vi "Pyro.vi"() -> ()   [LabVIEW 2013]
uses:
  <vilib>/Instr/_visa.llb/VISA Configure Serial Port (Instr).vi
panel:
  out "XY Graph":cluster{dbl[], i32[]}(graph)
  in  "wait":u32
  out "read buffer 3":string
  in  "CUSTOM COMMAND":string(combo)
  in  "Enable Termination\nChar (T)":bool=TRUE
  in  "termination char\n(0xA = '\\n' = LF)":u8=10 format="%.0x"
  in  "timeout (10sec)":u32=10000
  in  "flow control (0:none)":u16(ring) items=["None", "XON/XOFF", "RTS/CTS", "XON/XOFF & RTS/CTS", "DTR/DSR", "XON/XOFF & DTR/DSR"]
  in  "stop bits (10: 1 bit)":u16(ring)=10 items=["1.0"=10, "1.5"=15, "2.0"=20]
  in  "data bits (8)":u16=8 min=5 max=8 step=1
  in  "parity (0:none)":enum16{"None", "Odd", "Even", "Mark", "Space"}(ring)=enum."Even"
  in  "baud rate (9600)":u32=19200
  in  "VISA resource name":refnum<visa-resource-name>="COM3"
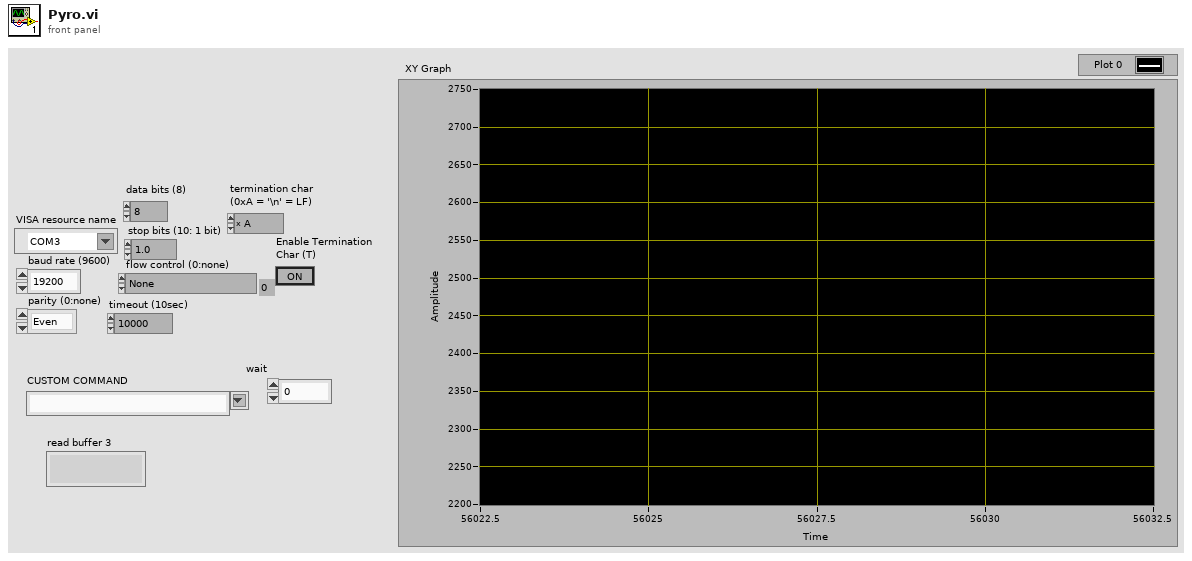
[diagram p1: front panel]
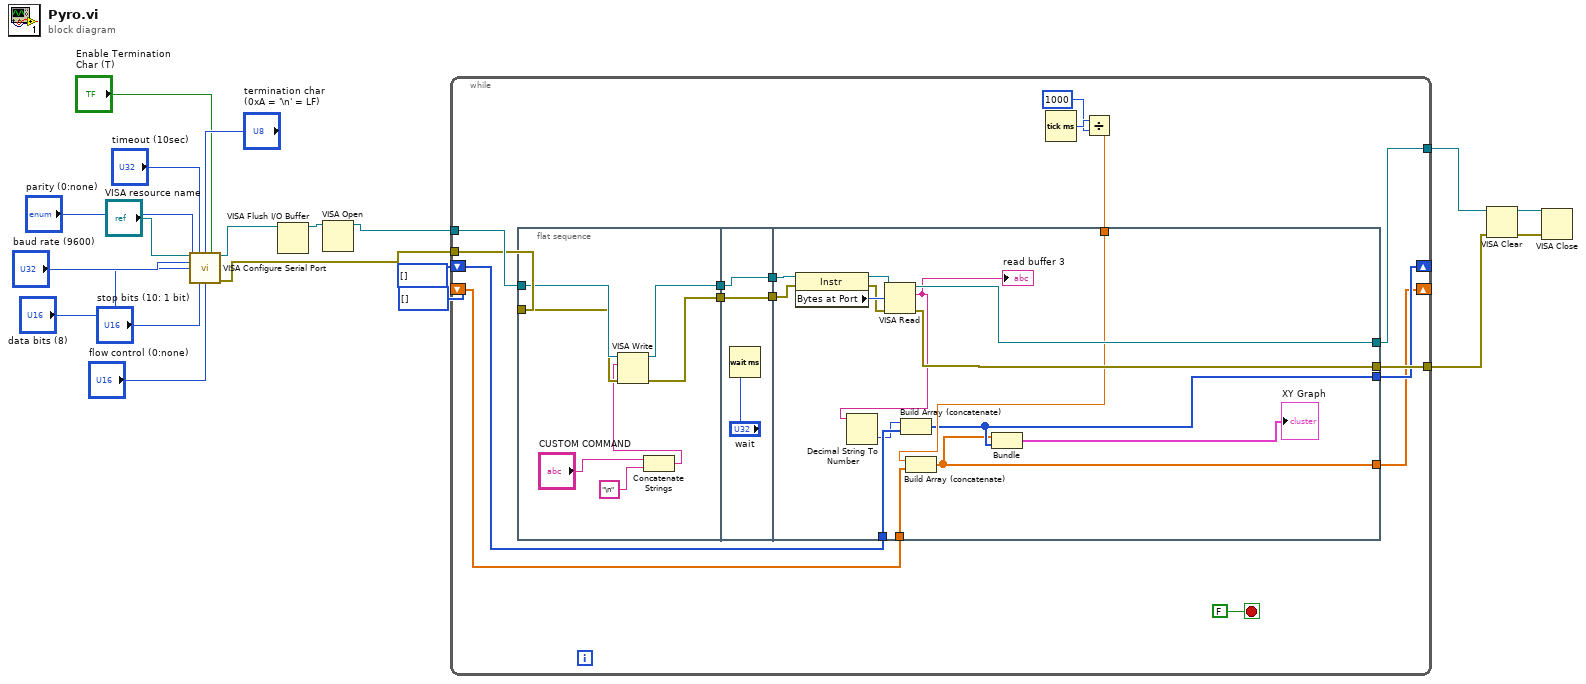
[diagram p0: block diagram]
diagram:
  n1 = call-poly "VISA Configure Serial Port"("VISA resource name"="VISA resource name", "timeout (10sec)"="timeout (10sec)", "termination char\n(0xA = '\\n' = LF)"="termination char\n(0xA = '\\n' = LF)", "Enable Termination\nChar (T)"="Enable Termination\nChar (T)", "baud rate (9600)"="baud rate (9600)", "data bits (8)"="data bits (8)", "parity (0:none)"="parity (0:none)", "stop bits (10: 1 bit)"="stop bits (10: 1 bit)", "flow control (0:none)"="flow control (0:none)") -> ("VISA resource name out"=w14:refnum<visa-resource-name>, "error out"=w13:errorcluster)  [unwired: 5 in]
  n2 = VISA Flush I/O Buffer(VISA resource name=w14) -> (VISA resource name out=w15:refnum<visa-resource-name>)  [unwired: 2 in, 1 out]
  n3 = VISA Open(VISA resource name=w15) -> (VISA resource name=w16:refnum<visa-resource-name>)  [unwired: 4 in, 1 out]
  n4 = while {
    tunnel: w16 -> [w28]
    shift-right: [w21] -> _
    shift-left: i32[] [] -> [w24]
    shift-right: [w20] -> _
    shift-left: u32[] [] -> [w22]
    tunnel: w13 -> [w27]
    tunnel: [w26] -> w3
    tunnel: [w25] -> w2
    stop <- FALSE stop-if-true
    n5 = flat-sequence {
      tunnel: [w42] -> w32
      tunnel: [w41] -> w31
      tunnel: w28 -> [w40]
      tunnel: w27 -> [w39]
      tunnel: w32 -> [w45]
      tunnel: w31 -> [w44]
      tunnel: [w45] -> w30
      tunnel: [w44] -> w29
      tunnel: w30 -> [w58]
      tunnel: w29 -> [w57]
      tunnel: [w55] -> w26
      tunnel: [w54] -> w25
      tunnel: w24 -> [w52]
      tunnel: w23 -> [w51]
      tunnel: w22 -> [w50]
      tunnel: [w48] -> w21
      tunnel: [w47] -> w20
      frame #0 {
        n6 = Concatenate Strings("CUSTOM COMMAND", "\n" ("string")) -> (w37:string)
        n7 = VISA Write(VISA resource name=w40, write buffer=w37, error in (no error)=w39) -> (VISA resource name out=w42:refnum<visa-resource-name>, error out=w41:errorcluster)  [unwired: 1 out]
      }
      frame #1 {
        n8 = Wait (ms)(milliseconds to wait="wait") -> ()  [unwired: 1 out]
      }
      frame #2 {
        n9 = property class="Instr"(reference=w58, error in=w57) -> (reference out=w59:refnum<visa-resource-name>, error out=w56:errorcluster, "Bytes at Port"=w60:u32)
        n10 = VISA Read(VISA resource name=w59, byte count=w60, error in (no error)=w56) -> (VISA resource name out=w55:refnum<visa-resource-name>, read buffer=w53:string, error out=w54:errorcluster)  [unwired: 1 out]
        "read buffer 3" <- w53
        n11 = Decimal String To Number(string=w53) -> (number=w46:i32)  [unwired: 2 in, 1 out]
        n12 = Build Array (concatenate)(w46, w52) -> (w48:i32[])
        n13 = Build Array (concatenate)(w51, w50) -> (w47:dbl[])
        n14 = Bundle(w47, w48) -> (→"XY Graph":cluster{dbl[], i32[]})  [unwired: 1 in]
      }
    }
    n15 = Tick Count (ms)() -> (millisecond timer value=w34:u32)
    n16 = Divide(x=w34, y=u32 1000) -> (x/y=w23:dbl)
  }
  n17 = VISA Clear(VISA resource name=w3, error in (no error)=w2) -> (VISA resource name out=w17:refnum<visa-resource-name>, error out=w1:errorcluster)
  n18 = VISA Close(VISA resource name=w17, error in (no error)=w1) -> ()  [unwired: 1 out]
